vi "Init.vi"(8 "error in":errorcluster, 10 "Session":string, 11 "SR3XXX HVPS in":refnum<class "SR3XXX HVPS.lvclass">) -> (0 "error out":errorcluster, 3 "SR3XXX HVPS out":refnum<class "SR3XXX HVPS.lvclass">)   [LabVIEW 2013, in "SR3XXX HVPS.lvclass"]
uses:
  SR3XXX HVPS.lvclass
  Reusable/Session APIs/Serial/Serial Session.lvclass
  Reusable/Session APIs/Serial/Typedefs/Msg Config.ctl
  Reusable/Session APIs/Serial/Serial Session.lvclass/Serial Session.ctl
  Base/Session HVPS.lvclass/Session HVPS.ctl
  Reusable/Session APIs/Serial/Public/Accessors/Write VISA Resource.vi
  Base/Write hSession.vi
  Reusable/Session APIs/Serial/Public/Configure Messaging.vi
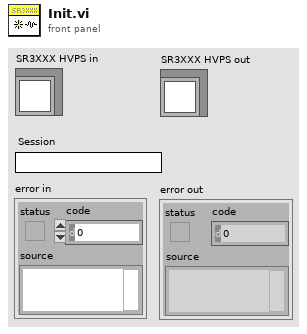
[diagram p1: front panel]
types:
  T1 = typedef "Serial Session.lvclass/Msg Config.ctl" = cluster{"sendEndEn":bool, "suppEnEnRd":bool, "termChar":u8, "EnTermChar":bool}
  T2 = typedef "Serial Session.lvclass/Session Handle.ctl" = refnum<data-value>
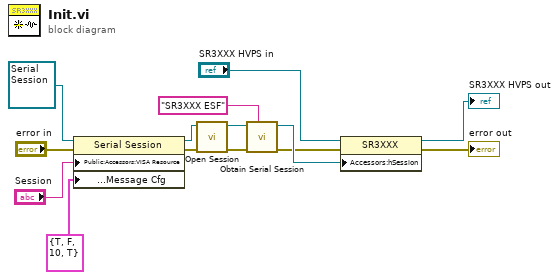
[diagram p0: block diagram]
diagram:
  n1 = property class="Serial Session"(reference=refnum<class "Serial Session.lvclass"> refnum ("Serial Session"), error in="error in", "Public:Accessors:VISA Resource"="Session", "Public:Configuration:Message Cfg"=T1 {"sendEndEn"=TRUE, "suppEnEnRd"=FALSE, "termChar"=10, "EnTermChar"=TRUE} ("Message Cfg")) -> (reference out=w10:refnum<class "Serial Session.lvclass">, error out=w9:errorcluster)
  n2 = call "Open Session.vi"("error in (no error)"=w9, "Serial Session in"=w10) -> ("error out"=w6:errorcluster, "Serial Session out"=w8:refnum<class "Serial Session.lvclass">)  [unwired: 8 in]
  n3 = call "Obtain Serial Session.vi"("Session Name ()"="SR3XXX ESF", "error in"=w6, "Serial Session in"=w8) -> ("error out"=w2:errorcluster, "hSerial"=w4:T2)  [unwired: 6 in, 1 out]
  n4 = property class="SR3XXX"(reference="SR3XXX HVPS in", error in=w2, "Accessors:hSession"=w4) -> (reference out=→"SR3XXX HVPS out":refnum<class "SR3XXX HVPS.lvclass">, error out=→"error out":errorcluster)
